vi "MetaTabs.vi"() -> ()   [LabVIEW 2024, in "UIs Handler.lvlib"]
uses:
  UIs Handler.lvlib
  Custom Controls/Control Alarms_Tab boolean.ctl
  Custom Controls/Control Logger_Tab boolean.ctl
  Custom Controls/Control PID_Tab boolean.ctl
  Custom Controls/Control PS_Tab boolean.ctl
  States.ctl
  <vilib>/Utility/file.llb/Application Directory.vi
panel:
  out "2D Picture":picture
  in  "Control":T1
  in  "PIDs":T2
  in  "Logger":T3
  in  "Alarm":T4
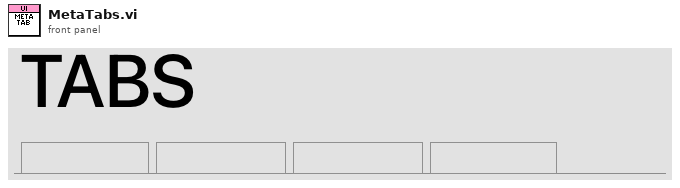
[diagram p1: front panel]
types:
  T1 = typedef "UIs Handler.lvlib/Control PS_Tab boolean.ctl" = bool
  T2 = typedef "UIs Handler.lvlib/Control PID_Tab boolean.ctl" = bool
  T3 = typedef "UIs Handler.lvlib/Control Logger_Tab boolean.ctl" = bool
  T4 = typedef "UIs Handler.lvlib/Control Alarms_Tab boolean.ctl" = bool
  T5 = typedef "UIs Handler.lvlib/States.ctl" = enum16{"Init", "Wait for Event", "Error", "Read Image", "Close"}
  T6 = typedef "UIs Handler.lvlib/Broadcast Events--cluster.ctl" = cluster{"Module Did Init":refnum<user-event>, "Status Updated":refnum<user-event>, "Error Reported":refnum<user-event>, "Module Did Stop":refnum<user-event>, "Update Module Execution Status":refnum<user-event>, "Update Data":refnum<user-event>}
  T7 = typedef "imagedata.ctl" = cluster{"image type":i32, "image depth":i32, "image":u8[], "mask":u8[], "colors":u32[], "Rectangle":cluster{"left":i16, "top":i16, "right":i16, "bottom":i16}}
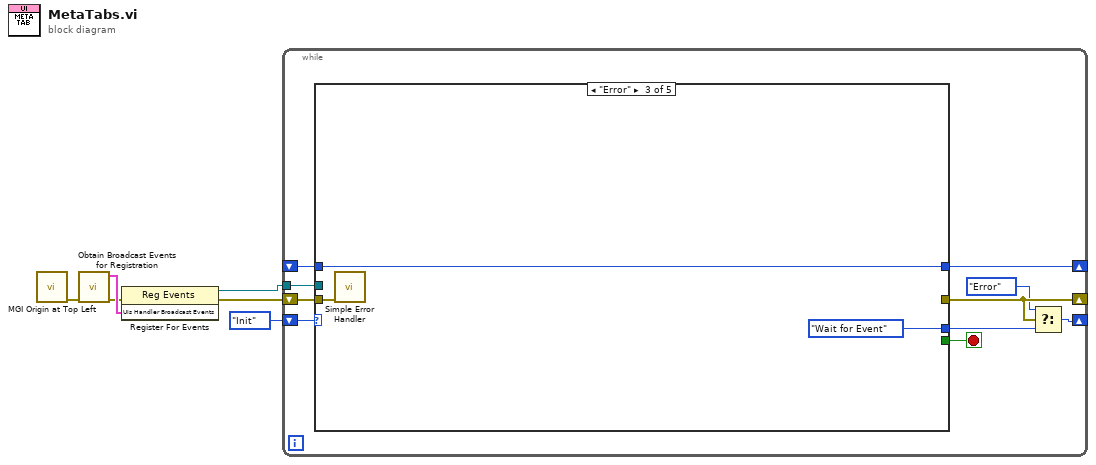
[diagram p0: block diagram]
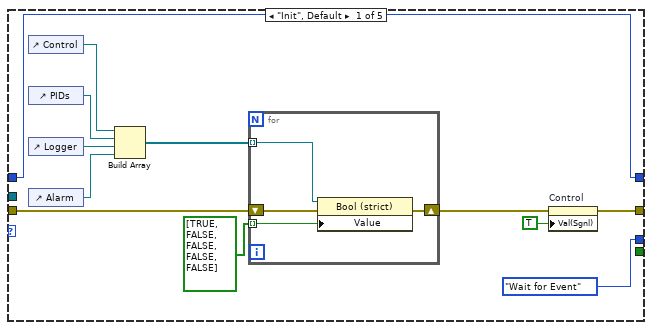
[diagram p2: hidden frame]
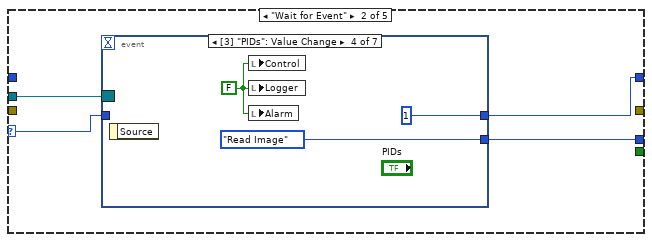
[diagram p3: hidden frame]
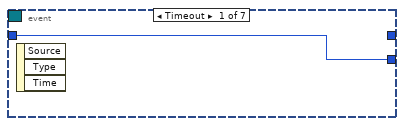
[diagram p4: hidden frame]
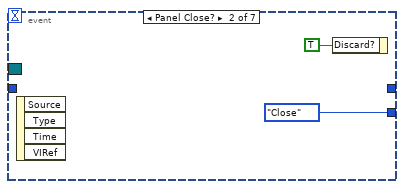
[diagram p5: hidden frame]
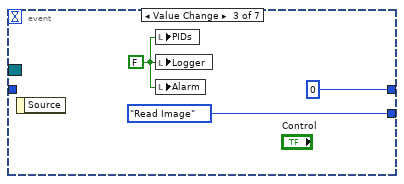
[diagram p6: hidden frame]
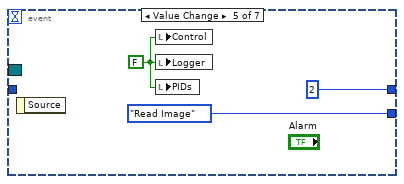
[diagram p7: hidden frame]
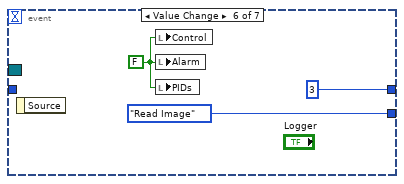
[diagram p8: hidden frame]
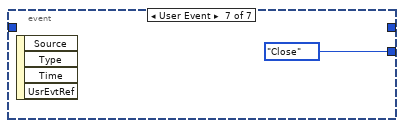
[diagram p9: hidden frame]
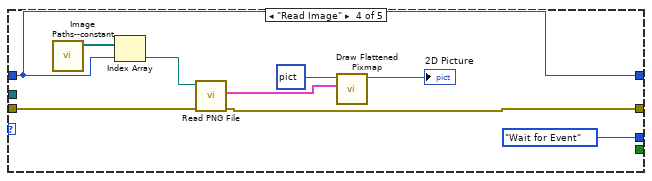
[diagram p10: hidden frame]
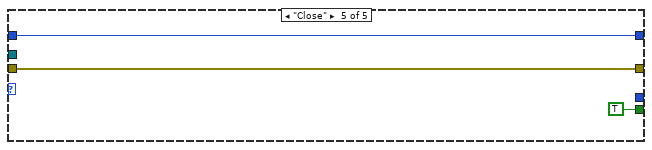
[diagram p11: hidden frame]
diagram:
  n1 = call <userlib>:"MGI Origin at Top Left.vi"() -> ("Error Out"=w3:errorcluster)  [unwired: 9 in, 1 out]
  n2 = call "Obtain Broadcast Events for Registration.vi"("error in"=w3) -> ("error out"=w4:errorcluster, "UIs Handler Broadcast Events"=w5:T6)  [unwired: 8 in, 1 out]
  n3 = register-events(error in=w4, w5) -> (reference out=w2:refnum<event-registration>, error out=w1:errorcluster)  [unwired: 1 in]
  n4 = while {
    shift-right: [w8] -> _
    shift-left: States."Init" ("States") -> [w16]
    shift-right: [w15] -> _
    shift-left: _ -> [w14]
    tunnel: w2 -> [w12]
    shift-right: [w10] -> _
    shift-left: w1 -> [w11]
    stop <- w13 stop-if-true
    n5 = case shown="\"Error\"" w16 {
      selector: w16 -> [_ w34 _ _ _]
      tunnel: [States."Wait for Event" ("States") w35 States."Wait for Event" ("States") States."Wait for Event" ("States") _] -> w9
      tunnel: [w21 w36 w54 w57 w67] -> w15
      tunnel: w14 -> [w21 _ w54 w57 w67]
      tunnel: [_ _ _ _ TRUE] -> w13
      tunnel: w12 -> [_ w33 _ _ _]
      tunnel: w11 -> [w18 _ w53 w60 w65]
      tunnel: [w17 _ _ w59 w65] -> w10
      frame "Init", Default {
        n6 = control-ref of="Control"() -> (w24:refnum<vi>)
        n7 = control-ref of="PIDs"() -> (w25:refnum<vi>)
        n8 = control-ref of="Logger"() -> (w26:refnum<vi>)
        n9 = control-ref of="Alarm"() -> (w27:refnum<vi>)
        n10 = Build Array(w24, w25, w26, w27) -> (w28:refnum<vi>[])
        n11 = for {
          tunnel: w28 -> [w32] mode=indexing
          tunnel: T4[] [TRUE, FALSE, FALSE, FALSE, FALSE] ("Value") -> [w31] mode=indexing
          shift-right: [w29] -> w20
          shift-left: w18 -> [w30]
          n12 = property class="Bool (strict)"(reference=w32, error in=w30, "Value"=w31) -> (error out=w29:errorcluster)  [unwired: 1 out]
        }
        n13 = property on="Control" class="Bool (strict)"(error in=w20, "Val(Sgnl)"=T1 TRUE ("Value (Signaling)")) -> (error out=w17:errorcluster)  [unwired: 1 in, 1 out]
      }
      frame "Wait for Event" {
        n14 = event shown="[3] \"PIDs\": Value Change" {
          selector: w33 -> [_ _ _ _ _ _ _]
          dyn-events: _ -> [_ _ _ _ _ _ _]
          timeout: _ -> [_ _ _ _ _ _ _]
          tunnel: [_ _ 0 1 2 3 _] -> w36
          tunnel: [w37 States."Close" ("States") States."Read Image" ("States") States."Read Image" ("States") States."Read Image" ("States") States."Read Image" ("States") States."Close" ("States")] -> w35
          tunnel: w34 -> [w37 _ _ _ _ _ _]
          event Timeout {
            n15 = event-data() -> ()  [unwired: 1 in, 3 out]
          }
          event Panel Close? {
            n16 = event-data() -> ()  [unwired: 1 in, 4 out]
            n17 = event-data("Discard?"=TRUE) -> ()  [unwired: 1 in, 1 out]
          }
          event Value Change {
            w42 = T2 FALSE ("PIDs")
            n18 = event-data() -> ()  [unwired: 1 in, 1 out]
            n19 = local write "PIDs"(w42) -> ()
            n20 = local write "Logger"(w42) -> ()
            n21 = local write "Alarm"(w42) -> ()
          }
          event Value Change {
            w45 = T2 FALSE ("PIDs")
            n22 = event-data() -> ()  [unwired: 1 in, 1 out]
            n23 = local write "Control"(w45) -> ()
            n24 = local write "Logger"(w45) -> ()
            n25 = local write "Alarm"(w45) -> ()
          }
          event Value Change {
            w48 = T2 FALSE ("PIDs")
            n26 = event-data() -> ()  [unwired: 1 in, 1 out]
            n27 = local write "Control"(w48) -> ()
            n28 = local write "Logger"(w48) -> ()
            n29 = local write "PIDs"(w48) -> ()
          }
          event Value Change {
            w51 = T2 FALSE ("PIDs")
            n30 = event-data() -> ()  [unwired: 1 in, 1 out]
            n31 = local write "Control"(w51) -> ()
            n32 = local write "Alarm"(w51) -> ()
            n33 = local write "PIDs"(w51) -> ()
          }
          event User Event {
            n34 = event-data() -> ()  [unwired: 1 in, 4 out]
          }
        }
      }
      frame "Error" {
        n35 = call <vilib>:"Simple Error Handler.vi"("error in (no error)"=w53) -> ()  [unwired: 4 in, 5 out]
      }
      frame "Read Image" {
        n36 = call "Image Paths--constant.vi"() -> ("Array"=w58:path[])  [unwired: 11 in]
        n37 = Index Array(array=w58, index=w57) -> (element=w56:path)
        n38 = call <vilib>:"Read PNG File.vi"("error in (no error)"=w60, "path to PNG file"=w56) -> ("error out"=w59:errorcluster, "image data"=w64:T7)  [unwired: 7 in, 1 out]
        n39 = call <vilib>:"Draw Flattened Pixmap.vi"("image data"=w64, "picture"=picture data[5B]) -> ("new picture"=→"2D Picture":picture)  [unwired: 7 in]
      }
      frame "Close" {
      }
    }
    n40 = Select(t=States."Error", s=w10, f=w9) -> (s? t:f=w8:T5)
  }
